vi "AntiBurn.vi"(5 "AllowedEncoderError":dbl=25.0 format="%#_13g", 7 "AllowedTimeDeviation":dbl=2.4 format="%#_13g", 8 "error in":errorcluster, 9 "MaxCurrent":dbl, 10 "MotorSetpoint":dbl, 11 "CAN Talon SRX Ref":T1={"DeviceStatus"={"status"=FALSE, "code"=0, "source"=""}, "Type"=enum."PWM", "PWM"={"PWM Channel"=enum."PWM 1", "DeadBand"={"Name"="", "maxPositivePwm"=0, "minPositivePwm"=0, "centerPwm"=0, "maxNegativePwm"=0, "minNegativePwm"=0, "angularRange"=0}}, "CAN"={"Device Number"=0, "Control Mode"=enum."Percent VBus", "Semaphore"=refnum, "Max Vout"=12.0, "TalonSRX Control Mode"=enum."Percent VBus"}, "Invert"=FALSE}) -> (0 "error out":errorcluster, 1 "TimeOfLastChange":timestamp=timestamp(3512669090.758719 s since 1904-01-01), 2 "MotorSetpointOut":dbl, 3 "MotorControlDevRef":T1={"DeviceStatus"={"status"=FALSE, "code"=0, "source"=""}, "Type"=enum."PWM", "PWM"={"PWM Channel"=enum."Invalid", "DeadBand"={"Name"="", "maxPositivePwm"=0, "minPositivePwm"=0, "centerPwm"=0, "maxNegativePwm"=0, "minNegativePwm"=0, "angularRange"=0}}, "CAN"={"Device Number"=0, "Control Mode"=enum."Percent VBus", "Semaphore"=refnum, "Max Vout"=12.0, "TalonSRX Control Mode"=enum."Percent VBus"}, "Invert"=FALSE})   [LabVIEW 2015]
uses:
  <vilib>/Rock Robotics/WPI/MotorControl/WPI_MotorControlDeviceRef.ctl
  <vilib>/Rock Robotics/WPI/MotorControl/WPI_MotorControlType.ctl
  <vilib>/Rock Robotics/SystemInterfaces/DIO/FPGA_DIOPWMChannel.ctl
  <vilib>/Rock Robotics/WPI/PWM/WPI_PWMDeadband.ctl
  <vilib>/Rock Robotics/WPI/CAN/Jaguar/SubVIs/WPI_CANJaguar_ControlMode.ctl
  <vilib>/Rock Robotics/WPI/CAN/TalonSRX/WPI_CANTalonSRX_APIControlMode.ctl
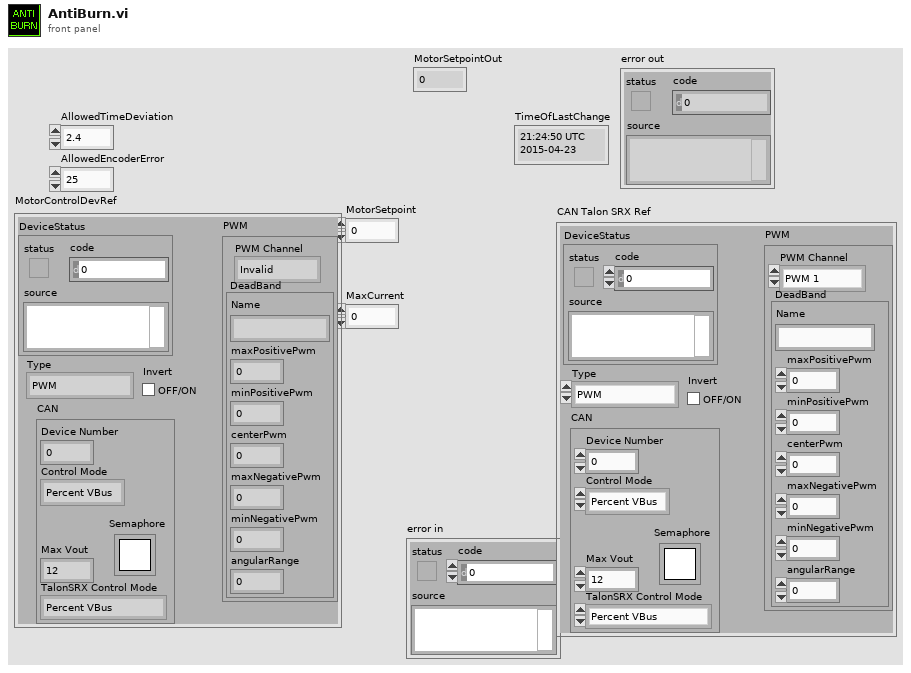
[diagram p1: front panel]
types:
  T1 = typedef "WPI_MotorControlDeviceRef.ctl" = cluster{"DeviceStatus":errorcluster, "Type":T2, "PWM":cluster{"PWM Channel":T3, "DeadBand":T4}, "CAN":cluster{"Device Number":u8, "Control Mode":T5, "Semaphore":T6, "Max Vout":dbl, "TalonSRX Control Mode":T7}, "Invert":bool}
  T2 = typedef "WPI_MotorControlType.ctl" = enum16{"PWM", "CAN", "CANTalonSRX"}
  T3 = typedef "FPGA_DIOPWMChannel.ctl" = enum8{"PWM 0", "PWM 1", "PWM 2", "PWM 3", "PWM 4", "PWM 5", "PWM 6", "PWM 7", "PWM 8", "PWM 9", "PWM MXP 0", "PWM MXP 1", "PWM MXP 2", "PWM MXP 3", "PWM MXP 4", "PWM MXP 5", "PWM MXP 6", "PWM MXP 7", "PWM MXP 8", "PWM MXP 9", "Invalid"}
  T4 = typedef "WPI_PWMDeadband.ctl" = cluster{"Name":string, "maxPositivePwm":i32, "minPositivePwm":i32, "centerPwm":i32, "maxNegativePwm":i32, "minNegativePwm":i32, "angularRange":u16}
  T5 = typedef "WPI_CANJaguar_ControlMode.ctl" = enum8{"Percent VBus", "Current", "Speed", "Position", "Voltage"}
  T6 = typedef "Semaphore RefNum" = refnum<k1>
  T7 = typedef "WPI_CANTalonSRX_APIControlMode.ctl" = enum8{"Percent VBus", "Speed", "Position", "Slave", "Unchanged / Invalid", "Voltage Compensation", "Current", "Motion Profile"}
  T8 = typedef "WPI_CANTalonSRX_GlobalStatus.ctl" = cluster{"Applied Throttle":dbl, "Module Enabled":bool, "CAN Error":errorcluster, "Closed Loop Error":dbl, "Forward Limit Switch Closed":bool, "Reverse Limit Switch Closed":bool, "Sensor Position":dbl, "Sensor Velocity":dbl, "Current":dbl, "Sticky Fault - Over Temp":bool, "Sticky Fault - Under Voltage":bool, "Sticky Fault - Forward Limit":bool, "Sticky Fault - Reverse Limit":bool, "Sticky Fault - Forward Soft Limit":bool, "Sticky Fault - Reverse Soft Limit":bool, "Brake is Enabled":bool, "Encoder Position":dbl, "Encoder Velocity":dbl, "Encoder Index Count":dbl, "Encoder A Pin State":bool, "Encoder B Pin State":bool, "Encoder Index Pin State":bool, "Analog In":dbl, "Analog In Velocity":dbl, "Temperature (C)":dbl, "Battery Voltage":dbl, "Control 5 Is Supported":bool, "Current Profile Slot Select":dbl, "Pos Div 8":bool, "Vel Div 4":bool, "Pulse Width Position":i32, "Pulse Width Velocity":i32, "Pulse Width Rise To Rise (us)":i32, "Pulse Width Rise To Fall (us)":i32, "Mot Prof Active Is Under Run":bool, "Mot Prof Active Has Under Run":bool, "Mot Prof Active Is Last":bool, "Mot Prof Active Velocity Only":bool, "Mot Prof Active Is Valid":bool, "Mot Prof Buffer Is Full":bool, "Mot Prof Active Profile Slot Select":i32, "Mot Prof NextID":i32, "Mot Prof Count":i32, "Mot Prof Active Velocity":dbl, "Mot Prof Active Position":dbl, "Mot Prof Output Enable":i32}
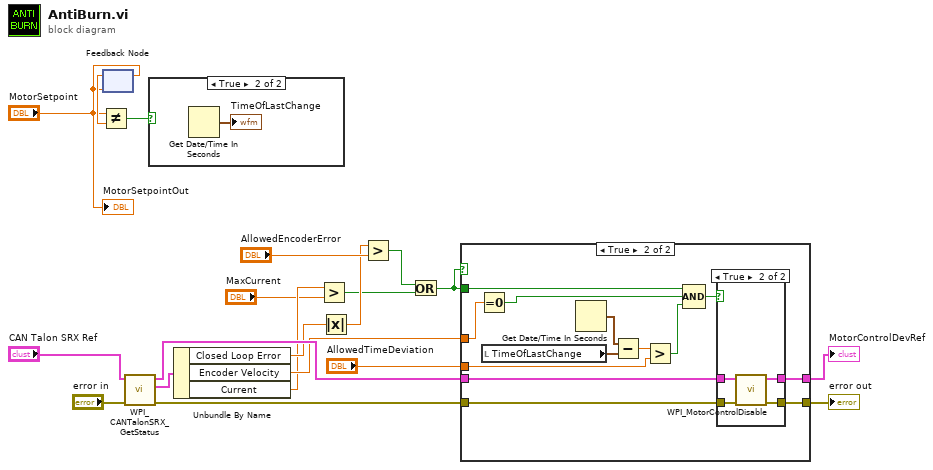
[diagram p0: block diagram]
diagram:
  n1 = feedback #1("MotorSetpoint") -> (w20:dbl)
  n2 = Not Equal?(x="MotorSetpoint", y=w20) -> (x != y?=w19:bool)
  n3 = feedback-in #1("MotorSetpoint") -> ()
  n4 = call <vilib>:"WPI_CANTalonSRX_GetStatus.vi"("error in (no error)"="error in", "CAN Talon SRX Ref"="CAN Talon SRX Ref") -> ("error out"=w18:errorcluster, "Talon SRX Status"=w14:T8, "CAN Talon SRX Ref"=w17:T1)  [unwired: 7 in]
  n5 = case shown="True" w19 {
    frame False {
    }
    frame True {
      n6 = Get Date/Time In Seconds() -> (seconds since 1Jan1904=→"TimeOfLastChange":timestamp)
    }
  }
  n7 = Unbundle By Name(w14) -> ("Closed Loop Error"=w15:dbl, "Encoder Velocity"=w16:dbl, "Current"=w10:dbl)
  n8 = Greater?(x=w10, y="MaxCurrent") -> (0:w9:bool)
  n9 = Absolute Value(x=w15) -> (abs(x)=w11:dbl)
  n10 = Greater?(x=w11, y="AllowedEncoderError") -> (0:w8:bool)
  n11 = Or(x=w8, y=w9) -> (x .or. y?=w7:bool)
  n12 = case shown="True" w7 {
    tunnel: w7 -> [_ w30]
    tunnel: w16 -> [_ w36]
    tunnel: w17 -> [w22 w35]
    tunnel: w18 -> [w23 w34]
    tunnel: "AllowedTimeDeviation" -> [_ w26]
    tunnel: [w23 w25] -> w3
    tunnel: [w22 w24] -> w2
    frame False {
    }
    frame True {
      n13 = Equal To 0?(x=w36) -> (x = 0?=w29:bool)
      n14 = local read "TimeOfLastChange"() -> (w32:timestamp)
      n15 = Get Date/Time In Seconds() -> (seconds since 1Jan1904=w33:timestamp)
      n16 = Subtract(x=w33, y=w32) -> (x-y=w31:dbl)
      n17 = Greater?(x=w31, y=w26) -> (0:w28:bool)
      n18 = Compound Arithmetic op=AND(w30, w29, w28) -> (w27:bool)
      n19 = case shown="True" w27 {
        tunnel: w35 -> [w37 w42]
        tunnel: w34 -> [w38 w41]
        tunnel: [w38 w40] -> w25
        tunnel: [w37 w39] -> w24
        frame False {
        }
        frame True {
          n20 = call <vilib>:"WPI_MotorControlDisable.vi"("error in (no error)"=w41, "MotorControlDevRef"=w42) -> ("error out"=w40:errorcluster, "MotorControlDevRef"=w39:T1)  [unwired: 8 in]
        }
      }
    }
  }
  "error out" <- w3
  "MotorControlDevRef" <- w2
  "MotorSetpointOut" <- "MotorSetpoint"
